vi "Reset_resultbackground.vi"(8 "error in (no error)":errorcluster, 11 "appended array":refnum<vi>[](array[refnum])) -> (0 "error out":errorcluster)   [LabVIEW 2021]
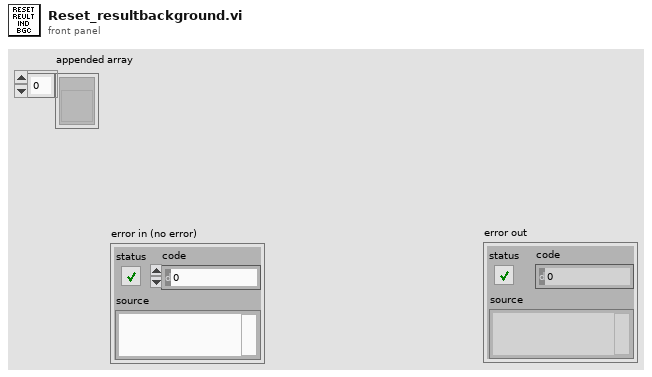
[diagram p1: front panel]
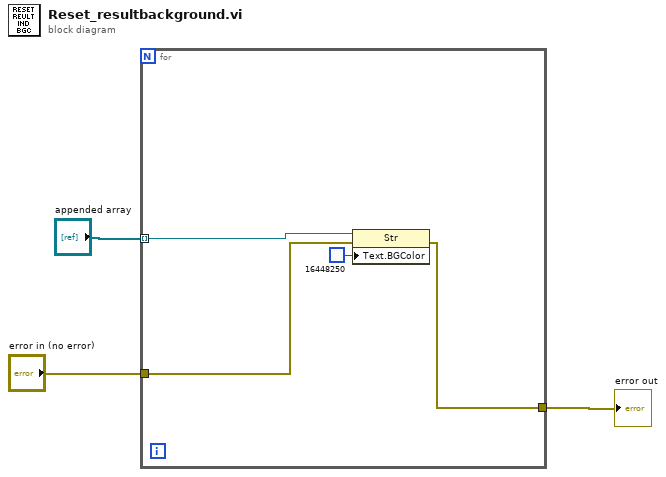
[diagram p0: block diagram]
diagram:
  n1 = for {
    tunnel: "appended array" -> [w7] mode=indexing
    tunnel: "error in (no error)" -> [w5]
    tunnel: [w4] -> w1
    n2 = property class="Str"(reference=w7, error in=w5, "Text.BGColor"=u32 16448250 ("Text.Text Colors:BG Color")) -> (error out=w4:errorcluster)  [unwired: 1 out]
  }
  "error out" <- w1
